vi "MasterAcquisitionFile_DALSA_IOS_MultiWavelength.vi"() -> ()   [LabVIEW 2020]
uses:
  <vilib>/vision/driver/IMAQdx.llb/IMAQdx Acquisition Mode.ctl
  <vilib>/vision/driver/IMAQdx.llb/IMAQdx Camera Control Mode.ctl
  <vilib>/userDefined/High Color/IMAQdx.ctl
  <vilib>/vision/driver/IMAQdx.llb/IMAQdx Buffer Number Mode.ctl
  <vilib>/DAQmx/write.llb/DAQmx Write (Digital 1D Wfm NChan NSamp).vi
  <vilib>/DAQmx/write.llb/DAQmx Write (Digital Bool 1Line 1Point).vi
  <vilib>/DAQmx/read.llb/DAQmx Read (Analog 1D Wfm NChan NSamp).vi
  <vilib>/Waveform/DWDTOps.llb/DWDT Digital to Boolean Array.vi
  <vilib>/DAQmx/create/channels.llb/DAQmx Create Channel (CO-Pulse Generation-Frequency).vi
  <vilib>/DAQmx/configure/timing.llb/DAQmx Timing (Implicit).vi
  <vilib>/DAQmx/create/channels.llb/DAQmx Create Channel (AI-Voltage-Basic).vi
  <vilib>/DAQmx/configure/timing.llb/DAQmx Timing (Sample Clock).vi
  <vilib>/DAQmx/configure/trigger.llb/DAQmx Start Trigger (Digital Edge).vi
  <vilib>/DAQmx/create/channels.llb/DAQmx Create Channel (DO-Digital Output).vi
  <vilib>/Waveform/DWDTOps.llb/DWDT Boolean Array to Digital.vi
  <vilib>/Waveform/DWDTOps.llb/DWDT Uncompress Digital.vi
  <vilib>/DAQmx/miscellaneous.llb/DAQmx Fill In Error Info.vi
  <vilib>/vision/driver/NI_Vision_Acquisition_Software.lvlib
  <resource>/objmgr/imaqdx.rc
  <resource>/objmgr/daqmx.rc
panel:
  out "LED":bool
  out "Auditory":bool
  out "RPad":bool
  out "LPad":bool
  out "Finished":bool
  in  "Generate Stimuli":bool=TRUE
  in  "Sol Stim Parameters":cluster{"Fs":dbl, "Samples":dbl}
  in  "LED Stim Parameters":cluster{"Fs":dbl, "Samples":dbl}
  in  "Sol Duty Cycle (%)":dbl=50.0
  in  "Sol Freq":dbl=1.0
  in  "Sol Dur (s)":dbl=1.0
  in  "LED Duty Cycle (%)":dbl=10.0
  in  "LED Freq":dbl=10.0
  in  "LED Dur (s)":dbl=2.0
  out "Stimulus Order":digitalwaveform[](graph)=[{"t0"=timestamp(0 s since 1904-01-01), "dt"=5e-05, "Y"={"transitions"=[], "data"=array18001000x1[18001000 elements]}}, {"t0"=timestamp(0 s since 1904-01-01), "dt"=5e-05, "Y"={"transitions"=[], "data"=array18001000x1[18001000 elements]}}, {"t0"=timestamp(0 s since 1904-01-01), "dt"=5e-05, "Y"={"transitions"=[], "data"=array18001000x1[18001000 elements]}}, {"t0"=timestamp(0 s since 1904-01-01), "dt"=5e-05, "Y"={"transitions"=[], "data"=array18001000x1[18001000 elements]}}]
  out "Solenoid Stim":digitalwaveform(graph)={"t0"=timestamp(0 s since 1904-01-01), "dt"=5e-05, "Y"={"transitions"=[], "data"=array100000x1[100000 elements]}}
  in  "Trial Offset (s)":dbl=15.0
  in  "Interstim (s)":dbl=30.0
  in  "Right Pad":dbl=1.0
  in  "Left Pad":dbl=1.0
  in  "Auditory":dbl=1.0
  in  "LED":dbl
  out "?":T1(plugin-control)
  out "?":T1(plugin-control)
  out "?":T1(plugin-control)
  out "?":T1(plugin-control)
  in  "stop":bool
  out "CBV Cam":bool
  out "Pupil Cam":bool
  out "Whisk Cam":bool
  out "Web Cam":bool
  out "Analog":bool
  out "Web Cam Fs":dbl(knob) scale=0.0..200.0
  out "CBV Cam Fs":dbl(knob) scale=0.0..200.0
  out "Whisk Cam Fs":dbl(knob) scale=0.0..200.0
  out "Last Whisk\nBuffer 2":u32=1590
  out "Pupil Cam Fs":dbl(knob) scale=0.0..200.0
  out "Dropped 2":u32(slide) caption="Pupil Cam" scale=0.0..99.0
  out "Dev1 Samples":i32
  in  "Dev1 Analog Channels":string[](array[string])=["Cortical_LH", "Force_Sensor", "LPadSol", "RPadSol", "AudSol", "Hippocampus", "EMG", "Cortical_RH", "OptoLED"]
  in  "Analog Acquisition":cluster{"Analog Fs":u16}={"Analog Fs"=20000} {"Analog Fs" format="%0.0f"}
  in  "Sampling Rates":T2={"Web Cam Fs"=30, "Whisk Cam Fs"=150, "Pupil Cam Fs"=30, "CBV Cam Fs"=30}
  out "Notes Size":i32=8
  out "Notes Reversed":string[](array[string])=["Experimenter", "Animal ID", "Hemisphere", "Solenoid PSI", "Isoflurane time", "Session ID", "Amplifier Gain", "LED power (mW)"]
  out "Notes Array":string[](array[string])=["LED power (mW)", "Amplifier Gain", "Session ID", "Isoflurane time", "Solenoid PSI", "Hemisphere", "Animal ID", "Experimenter"]
  in  "Notes:":T3={"Experimenter"="Kevin", "Animal ID"="T305", "Hemisphere"="Both", "Solenoid PSI"="10", "Isoflurane time"="1325", "Session ID"="Imaging Session Four", "Amplifier Gain"="10000", "LED power (mW)"="10"}
  in  "Target Path":path=path "D:/SG06/Imaging Session 4 - 28 July 2022" caption="Final Save Location"
  out "Dropped":u32(slide) caption="Whisk Cam" scale=0.0..999.0
  out "Filename":string="220728_13_37_51"
  out "CBV Camera":bool
  out "Time Elapsed (Min)":cluster{dbl, dbl}(slide)={15.0, 0.0} scale=0.0..15.0 scale format="%#_2g"
  in  "Time (min)":dbl(knob)=15.0 min=0.5 max=20.0 step=0.5 scale=0.0..20.0 scale format="%#_2g"
  in  "Temp Path":path=path "D:/LabVIEW Streamed Data" caption="Temporary Path for Streamed Data"
  out "Last CBV\nBuffer":i32=1590
  out "Last Whisk\nBuffer":u32=7953
  # "Dropped Frames"
  # "Stimuli"
  # "LPAD"
  # "RPAD"
  # "AUD"
  # "LED"
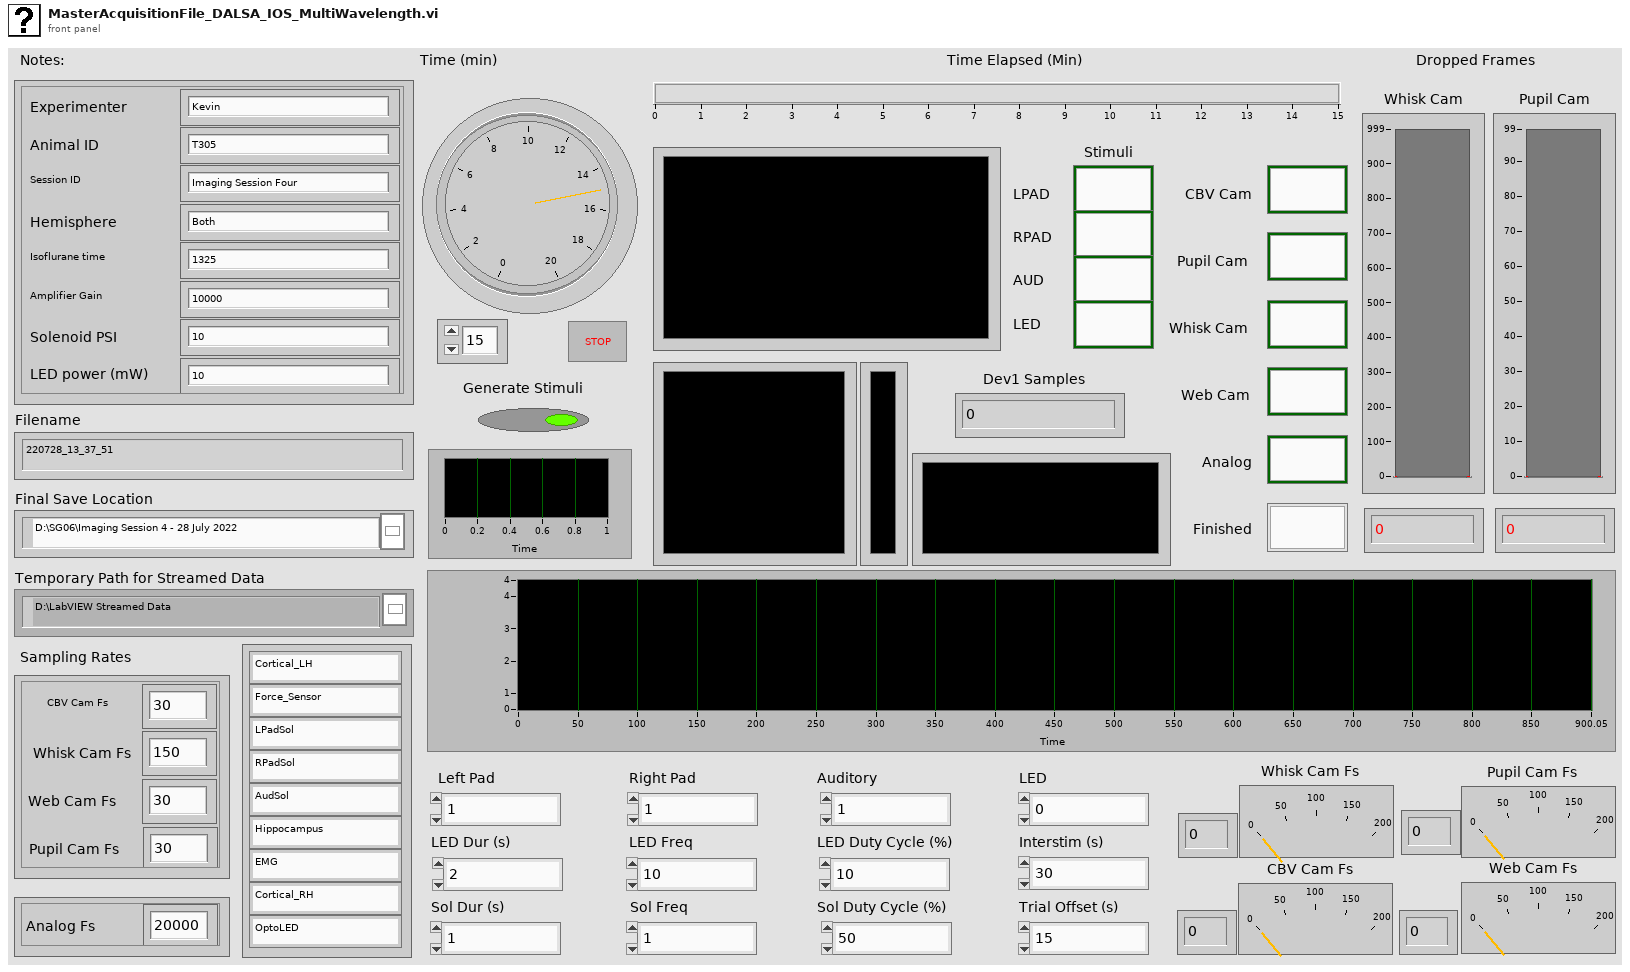
[diagram p1: front panel]
types:
  T1 = typedef "IMAQ Image.ctl" = refnum<image>
  T2 = cluster{"Web Cam Fs":u16, "Whisk Cam Fs":u16, "Pupil Cam Fs":u16, "CBV Cam Fs":u16}
  T3 = cluster{"Experimenter":string, "Animal ID":string, "Hemisphere":string, "Solenoid PSI":string, "Isoflurane time":string, "Session ID":string, "Amplifier Gain":string, "LED power (mW)":string}
  T4 = typedef "IMAQdx.ctl" = refnum<k21>
  T5 = enum16{"open", "replace", "create", "open or create", "replace or create", "replace or create with confirmation"}
  T6 = typedef "Image Type" = u32
  T7 = typedef "NI_Vision_Acquisition_Software.lvlib/IMAQdx Acquisition Mode.ctl" = enum32{"One Shot", "Continuous"}
  T8 = typedef "NI_Vision_Acquisition_Software.lvlib/IMAQdx Camera Control Mode.ctl" = enum32{"Controller", "Listener"}
  T9 = enum16{"open", "open or create", "create or replace", "create", "open (read-only)"}
  T10 = typedef "IMAQ AVI2 Refnum.ctl" = refnum<k20>
  T11 = enum16{"big-endian, network order", "native, host order", "little-endian"}
  T12 = typedef "NI_Vision_Acquisition_Software.lvlib/IMAQdx Buffer Number Mode.ctl" = enum32{"Next", "Last", "Buffer Number", "Every", "Last New"}
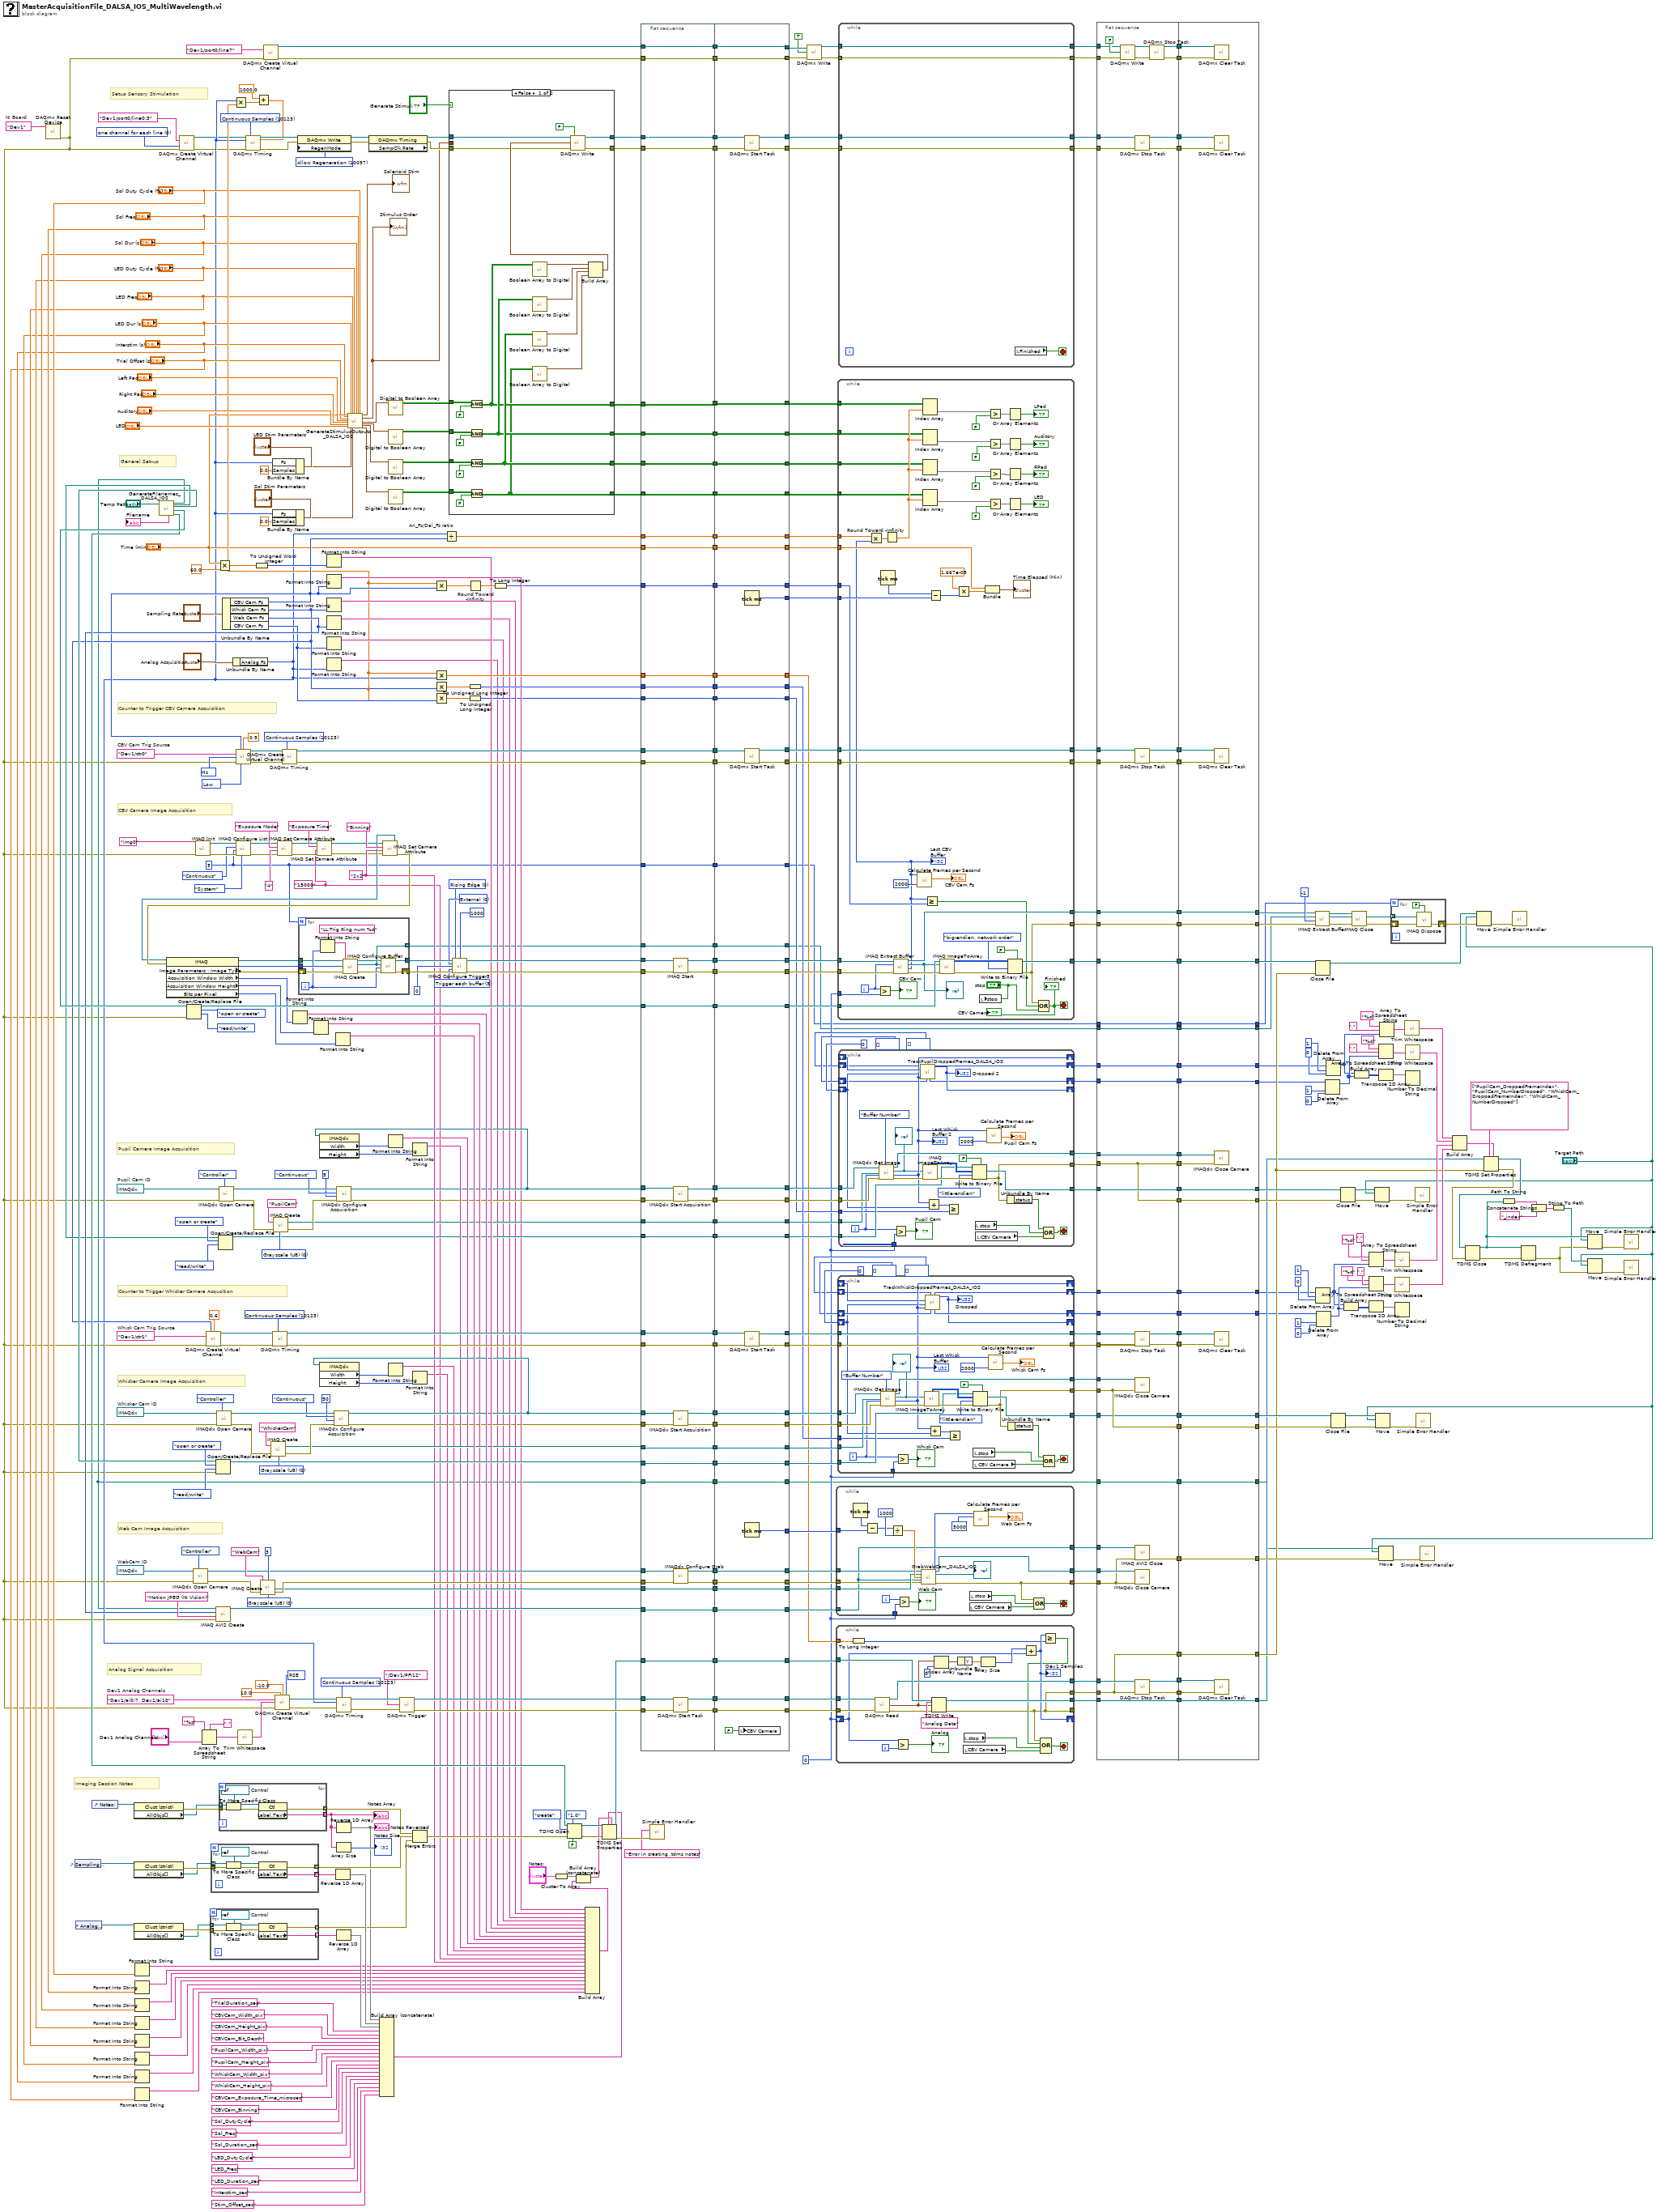
[diagram p0: block diagram]
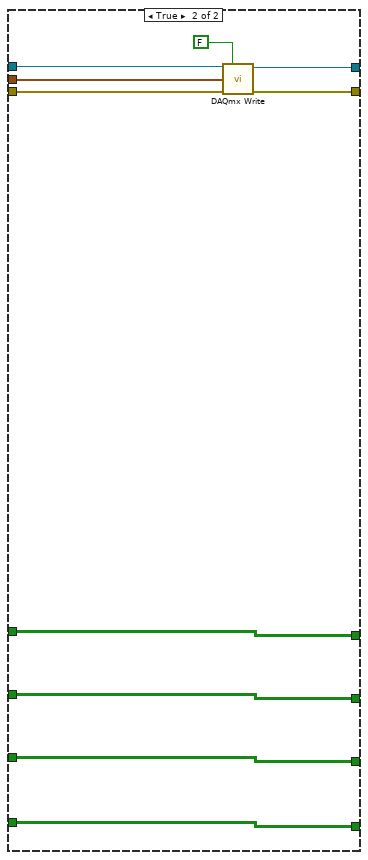
[diagram p2: hidden frame]
diagram:
  w2 = "15000" ("Exposure Time (microsec)")
  w129 = 10097 items=["Allow Regeneration"=10097, "Do Not Allow Regeneration"=10158] ("RegenMode")
  w130 = 10123 items=["Finite Samples"=10178, "Continuous Samples"=10123, "Hardware Timed Single Point"=12522] ("sample mode")
  w133 = 0 items=["one channel for each line", "one channel for all lines"] ("line grouping")
  w327 = tag "Dev1/ai0:7, Dev1/ai10"  # Dev1 Analog Channels
  w330 = T4 "cam3"  # WebCam ID
  w308 = T4 "cam1"  # Whisker Cam ID
  w484 = tag "Dev1/ctr1"  # Whisk Cam Trig Source
  w258 = T4 "cam2"  # Pupil Cam ID
  w95 = tag "Dev1/ctr0"  # CBV Cam Trig Source
  w261 = T6 0 items=["Grayscale (U8)", "Grayscale (I16)", "Grayscale (SGL)", "Complex (CSG)", "RGB (U32)", "HSL (U32)", "RGB (U64)", "Grayscale (U16)"] ("Image Type")
  w248 = "2x2" ("Attribute Value")
  w186 = 0
  w403 = 10123 items=["Finite Samples"=10178, "Continuous Samples"=10123, "Hardware Timed Single Point"=12522] ("sample mode")
  w406 = 10083 items=["default"=-1, "RSE"=10083, "NRSE"=10078, "Differential"=10106, "Pseudodifferential"=12529] ("input terminal configuration")
  w450 = T6 0 items=["Grayscale (U8)", "Grayscale (I16)", "Grayscale (SGL)", "Complex (CSG)", "RGB (U32)", "HSL (U32)", "RGB (U64)", "Grayscale (U16)"] ("Image Type")
  w466 = u32 0 items=["Rising Edge", "Falling Edge"] ("Trigger Polarity")
  w469 = u32 0 items=["External"=0, "RTSI"=1, "ISO In"=2, "Scaled Encoder"=5] ("Trigger Type")
  w460 = tag "Dev1"  # NI Board
  w461 = 10123 items=["Finite Samples"=10178, "Continuous Samples"=10123, "Hardware Timed Single Point"=12522] ("sample mode")
  w464 = 10373 items=["Hz"=10373] ("units")
  w465 = 10214 items=["High"=10192, "Low"=10214] ("idle state")
  w28 = u32 5 ("Number of Buffers")
  w467 = u32 3 items=["Disabled", "Trigger start of acquisition", "Trigger start of each buffer list", "Trigger each buffer", "Trigger each line (linescan)", "Trigger end of acquisition"] ("Action")
  w480 = 10123 items=["Finite Samples"=10178, "Continuous Samples"=10123, "Hardware Timed Single Point"=12522] ("sample mode")
  w487 = T6 0 items=["Grayscale (U8)", "Grayscale (I16)", "Grayscale (SGL)", "Complex (CSG)", "RGB (U32)", "HSL (U32)", "RGB (U64)", "Grayscale (U16)"] ("Image Type")
  # "General Set-up"
  # "Pupil Camera Image Acquisition"
  # "Whisker Camera Image Acquisition"
  # "Imaging Session Notes"
  # "Setup Sensory Stimulation"
  # "CBV Camera Image Acquisition"
  # "Counter to Trigger CBV Camera Acquisition"
  # "Counter to Trigger Whisker Camera Acqusition"
  # "Web Cam Image Acquisition"
  # "Analog Signal Acquisition"
  n1 = call <vilib>:"DAQmx Reset Device.vi"("device in"=w460) -> ("error out"=w20:errorcluster)  [unwired: 14 in]
  n2 = control-ref of="Sampling Rates"() -> (w336:refnum<vi>)
  n3 = control-ref of="Analog Acquisition"() -> (w335:refnum<vi>)
  n4 = control-ref of="Notes:"() -> (w357:refnum<vi>)
  n5 = property class="Clust (strict)"(reference=w357) -> (error out=w360:errorcluster, "AllObjs[]"=w277:refnum<vi>[])  [unwired: 1 in, 1 out]
  n6 = property class="Clust (strict)"(reference=w336) -> (error out=w355:errorcluster, "AllObjs[]"=w278:refnum<vi>[])  [unwired: 1 in, 1 out]
  n7 = property class="Clust (strict)"(reference=w335) -> (error out=w334:errorcluster, "AllObjs[]"=w276:refnum<vi>[])  [unwired: 1 in, 1 out]
  n8 = Format Into String("Sol Duty Cycle (%)") -> (resulting string=w163:string)  [unwired: 3 in, 1 out]
  n9 = Format Into String("Sol Freq") -> (resulting string=w162:string)  [unwired: 3 in, 1 out]
  n10 = Format Into String("Sol Dur (s)") -> (resulting string=w161:string)  [unwired: 3 in, 1 out]
  n11 = Format Into String("LED Duty Cycle (%)") -> (resulting string=w160:string)  [unwired: 3 in, 1 out]
  n12 = Format Into String("LED Freq") -> (resulting string=w159:string)  [unwired: 3 in, 1 out]
  n13 = Format Into String("LED Dur (s)") -> (resulting string=w158:string)  [unwired: 3 in, 1 out]
  n14 = Format Into String("Interstim (s)") -> (resulting string=w157:string)  [unwired: 3 in, 1 out]
  n15 = Format Into String("Trial Offset (s)") -> (resulting string=w156:string)  [unwired: 3 in, 1 out]
  n16 = call "GenerateFilenames_DALSA_IOS.vi"("path"="Temp Path") -> ("TDMS Path"=w352:path, "Dalsa Path"=w457:path, "Basler Path"=w453:path, "WebCam Path"=w22:path, "Analog file name"=→"Filename":string, "Basler2 Path"=w257:path)  [unwired: 3 in, 2 out]
  n17 = call-poly <vilib>:"DAQmx Create Virtual Channel.vi"("lines"=tag "Dev1/port0/line0:3", "line grouping"=w133, "error in"=w20) -> ("task out"=w132:refnum<k21>, "error out"=w131:errorcluster)  [unwired: 11 in]
  n18 = Open/Create/Replace File(file path (use dialog)=w457, error in=w20, operation (0:open)=T5."open or create", access (0:read/write)=enum16{"read/write", "read-only", "write-only"}."read/write") -> (refnum out=w407:refnum<file>)  [unwired: 2 in, 2 out]
  n19 = call <vilib>:"IMAQdx Open Camera.vi"("Camera Control Mode"=IMAQdx_Camera_Control_Mode."Controller", "error in"=w20, "Session In"=w330) -> ("error out"=w446:errorcluster, "Session Out"=w444:T4)  [unwired: 7 in]
  n20 = call <vilib>:"IMAQ Init.vi"("error in (no error)"=w20, "Interface Name"="img0") -> ("error out"=w478:errorcluster, "IMAQ Session Out"=w479:refnum<k11>)  [unwired: 8 out]
  n21 = Array To Spreadsheet String(delimiter (Tab)=",", array="Dev1 Analog Channels", 3:"%s" ("format string")) -> (spreadsheet string=w324:string)
  n22 = for {
    tunnel: [w499] -> w332 mode=indexing
    tunnel: w334 -> [w498]
    tunnel: [w496] -> w333 mode=indexing
    tunnel: w276 -> [w495] mode=indexing
    w500 = refnum<vi> refnum  # Control
    n23 = To More Specific Class(target class=w500, reference=w495, error in=w498) -> (specific class reference=w501:refnum<vi>, error out=w497:errorcluster)
    n24 = property class="Ctl"(reference=w501, error in=w497) -> (error out=w496:errorcluster, "Label.Text"=w499:string)  [unwired: 1 out]
  }
  n25 = for {
    tunnel: [w506] -> w356 mode=indexing
    tunnel: w355 -> [w505]
    tunnel: [w503] -> w342 mode=indexing
    tunnel: w278 -> [w502] mode=indexing
    w507 = refnum<vi> refnum  # Control
    n26 = To More Specific Class(target class=w507, reference=w502, error in=w505) -> (specific class reference=w508:refnum<vi>, error out=w504:errorcluster)
    n27 = property class="Ctl"(reference=w508, error in=w504) -> (error out=w503:errorcluster, "Label.Text"=w506:string)  [unwired: 1 out]
  }
  n28 = Open/Create/Replace File(file path (use dialog)=w453, error in=w20, operation (0:open)=T5."open or create", access (0:read/write)=enum16{"read/write", "read-only", "write-only"}."read/write") -> (refnum out=w423:refnum<file>)  [unwired: 2 in, 2 out]
  n29 = call <vilib>:"IMAQdx Open Camera.vi"("Camera Control Mode"=IMAQdx_Camera_Control_Mode."Controller", "error in"=w20, "Session In"=w308) -> ("error out"=w490:errorcluster, "Session Out"=w493:T4)  [unwired: 7 in]
  n30 = Multiply(x="Time (min)", y=60.0) -> (x*y=w173:dbl)
  n31 = Open/Create/Replace File(file path (use dialog)=w257, operation (0:open)=T5."open or create", access (0:read/write)=enum16{"read/write", "read-only", "write-only"}."read/write") -> (refnum out=w239:refnum<file>)  [unwired: 3 in, 2 out]
  n32 = call <vilib>:"IMAQdx Open Camera.vi"("Camera Control Mode"=IMAQdx_Camera_Control_Mode."Controller", "error in"=w20, "Session In"=w258) -> ("error out"=w264:errorcluster, "Session Out"=w267:T4)  [unwired: 7 in]
  n33 = for {
    tunnel: [w513] -> w359 mode=indexing
    tunnel: w360 -> [w512]
    tunnel: [w510] -> w343 mode=indexing
    tunnel: w277 -> [w509] mode=indexing
    w514 = refnum<vi> refnum  # Control
    n34 = To More Specific Class(target class=w514, reference=w509, error in=w512) -> (specific class reference=w515:refnum<vi>, error out=w511:errorcluster)
    n35 = property class="Ctl"(reference=w515, error in=w511) -> (error out=w510:errorcluster, "Label.Text"=w513:string)  [unwired: 1 out]
  }
  "Notes Array" <- w359
  n36 = Unbundle By Name("Sampling Rates") -> ("CBV Cam Fs"=w174:u16, "Whisk Cam Fs"=w228:u16, "Web Cam Fs"=w329:u16, "CBV Cam Fs"=w222:u16)
  n37 = call-poly <vilib>:"DAQmx Create Virtual Channel.vi"("frequency"=w228, "duty cycle"=0.6, "counter"=w484, "error in"=w20) -> ("task out"=w482:refnum<k21>, "error out"=w481:errorcluster)  [unwired: 10 in]
  n38 = call "IMAQ AVI2 Create"("error in (no error)"=w20, "Codec"="Motion JPEG (NI Vision)", "Frames Per Second"=w329, "AVI Path"=w22) -> ("AVI Refnum"=w436:T10)  [unwired: 6 in, 1 out]
  n39 = Unbundle By Name("Analog Acquisition") -> ("Analog Fs"=w146:u16)
  n40 = Multiply(x=w146, y=w173) -> (x*y=w106:dbl)
  n41 = call-poly <vilib>:"DAQmx Create Virtual Channel.vi"("frequency"=w174, "duty cycle"=0.9, "counter"=w95, "units"=w464, "error in"=w20, "idle state"=w465) -> ("task out"=w463:refnum<k21>, "error out"=w462:errorcluster)  [unwired: 8 in]
  n42 = call <vilib>:"IMAQ Configure List.vi"("Memory Location"=enum16{"System", "Onboard"}."System", "error in (no error)"=w478, "Number of buffers"=w28, "Continuous?"=enum16{"One-Shot", "Continuous"}."Continuous" ("Continuous ?"), "IMAQ Session In"=w479) -> ("error out"=w287:errorcluster, "IMAQ Session Out"=w285:refnum<k11>)  [unwired: 1 in, 4 out]
  n43 = call <vilib>:"Trim Whitespace.vi"("string"=w324) -> ("trimmed string"=w323:string)  [unwired: 1 in]
  n44 = To Unsigned Word Integer(number=w173) -> (unsigned 16bit integer=w319:u16)
  n45 = Add(x=1000.0, y=w106) -> (x+y=w104:dbl)
  n46 = call-poly <vilib>:"DAQmx Timing.vi"("task/channels in"=w132, "sample mode"=w130, "samples per channel"=w104, "rate"=w146, "error in"=w131) -> ("task out"=w126:refnum<k21>, "error out"=w125:errorcluster)  [unwired: 9 in]
  n47 = call "IMAQ Create"("Border Size"=3, "Image Name"="WebCam", "Image Type"=w450, "error in (no error)"=w446) -> ("New Image"=w443:T1, "error out"=w445:errorcluster)  [unwired: 1 in]
  n48 = call-poly <vilib>:"DAQmx Create Virtual Channel.vi"("lines"=tag "Dev1/port0/line7", "error in"=w20) -> ("task out"=w18:refnum<k21>, "error out"=w19:errorcluster)  [unwired: 12 in]
  n49 = call "IMAQ Create"("Image Name"="WhiskerCam", "Image Type"=w487, "error in (no error)"=w490) -> ("New Image"=w306:T1, "error out"=w488:errorcluster)  [unwired: 2 in]
  n50 = Bundle By Name(cluster="LED Stim Parameters", "Fs"=w146, "Samples"=0.0) -> (w179:cluster{"Fs":dbl, "Samples":dbl})
  n51 = Bundle By Name(cluster="Sol Stim Parameters", "Fs"=w146, "Samples"=0.0) -> (w180:cluster{"Fs":dbl, "Samples":dbl})
  n52 = call-poly <vilib>:"DAQmx Timing.vi"("task/channels in"=w482, "sample mode"=w480, "error in"=w481) -> ("task out"=w389:refnum<k21>, "error out"=w387:errorcluster)  [unwired: 11 in]
  n53 = call "IMAQ Create"("Image Name"="PupilCam", "Image Type"=w261, "error in (no error)"=w264) -> ("New Image"=w231:T1, "error out"=w262:errorcluster)  [unwired: 2 in]
  n54 = call-poly <vilib>:"DAQmx Create Virtual Channel.vi"("maximum value"=10.0, "minimum value"=-10.0, "input terminal configuration"=w406, "physical channels"=w327, "name to assign"=w323, "error in"=w20) -> ("task out"=w405:refnum<k21>, "error out"=w404:errorcluster)  [unwired: 8 in]
  n55 = call <vilib>:"IMAQ Set Camera Attribute.vi"("error in (no error)"=w287, "Attribute Value"="4", "Camera Attribute"="Exposure Mode", "IMAQ Session In"=w285) -> ("error out"=w4:errorcluster, "IMAQ Session Out"=w6:refnum<k11>)  [unwired: 4 in]
  n56 = call-poly <vilib>:"DAQmx Timing.vi"("task/channels in"=w463, "sample mode"=w461, "error in"=w462) -> ("task out"=w393:refnum<k21>, "error out"=w391:errorcluster)  [unwired: 11 in]
  n57 = property class="DAQmx Write"(reference=w126, error in=w125, "RegenMode"=w129) -> (reference out=w127:refnum<k21>, error out=w128:errorcluster)
  n58 = call <vilib>:"IMAQ Set Camera Attribute.vi"("error in (no error)"=w4, "Attribute Value"=w2, "Camera Attribute"="Exposure Time", "IMAQ Session In"=w6) -> ("error out"=w3:errorcluster, "IMAQ Session Out"=w5:refnum<k11>)  [unwired: 4 in]
  n59 = Format Into String(w319) -> (resulting string=w321:string)  [unwired: 3 in, 1 out]
  n60 = Format Into String(w174) -> (resulting string=w226:string)  [unwired: 3 in, 1 out]
  n61 = Format Into String(w228) -> (resulting string=w225:string)  [unwired: 3 in, 1 out]
  n62 = Format Into String(w329) -> (resulting string=w224:string)  [unwired: 3 in, 1 out]
  n63 = Format Into String(w222) -> (resulting string=w192:string)  [unwired: 3 in, 1 out]
  n64 = Format Into String(w146) -> (resulting string=w191:string)  [unwired: 3 in, 1 out]
  n65 = call <vilib>:"IMAQdx Configure Acquisition.vi"("error in"=w488, "Number of Buffers"=u32 50, "Continuous?"=IMAQdx_Acquisition_Mode."Continuous", "Session In"=w493) -> ("error out"=w199:errorcluster, "Session Out"=w307:T4)  [unwired: 6 in]
  n66 = property class="IMAQdx"(reference=w307) -> ("Width"=w318:u32, "Height"=w317:u32)  [unwired: 1 in, 2 out]
  n67 = Reverse 1D Array(array=w356) -> (reversed array=w346:string[])
  n68 = Reverse 1D Array(array=w359) -> (reversed array=w275:string[])
  "Notes Reversed" <- w275
  n69 = Array Size(array=w359) -> (size(s)=→"Notes Size":i32)
  n70 = Reverse 1D Array(array=w332) -> (reversed array=w331:string[])
  n71 = call <vilib>:"IMAQdx Configure Acquisition.vi"("error in"=w262, "Number of Buffers"=u32 5, "Continuous?"=IMAQdx_Acquisition_Mode."Continuous", "Session In"=w267) -> ("error out"=w241:errorcluster, "Session Out"=w232:T4)  [unwired: 6 in]
  n72 = property class="IMAQdx"(reference=w232) -> ("Width"=w256:u32, "Height"=w255:u32)  [unwired: 1 in, 2 out]
  n73 = call-poly <vilib>:"DAQmx Timing.vi"("task/channels in"=w405, "sample mode"=w403, "rate"=w146, "error in"=w404) -> ("task out"=w274:refnum<k21>, "error out"=w402:errorcluster)  [unwired: 10 in]
  n74 = call "GenerateStimulusOutputs_DALSA_IOS.vi"("Trial duration (min)"="Time (min)", "Rest duration(s)"="Interstim (s)", "trial offset (s)"="Trial Offset (s)", "Left Pad"="Left Pad", "Right Pad"="Right Pad", "Auditory"="Auditory", "LED"="LED", "LED Stim Duration (s)"="LED Dur (s)", "LED Stim Parameters"=w179, "LED Frequency"="LED Freq", "Sol Stim Parameters"=w180, "LED duty cycle (%)"="LED Duty Cycle (%)", "Sol Stim Duration (s)"="Sol Dur (s)", "Sol Frequency"="Sol Freq", "Sol Duty Cycle (%)"="Sol Duty Cycle (%)") -> ("Solenoid Stim Waveforms"=→"Solenoid Stim":digitalwaveform, "Stimulus Digital Outputs"=w107:digitalwaveform[], "Left Pad Out"=w137:digitalwaveform, "Auditory Out"=w136:digitalwaveform, "Right Pad Out"=w135:digitalwaveform, "LED Out"=w134:digitalwaveform)  [unwired: 7 in]
  "Stimulus Order" <- w107
  n75 = property class="DAQmx Timing" props=["SampClk.Rate"](reference=w127, error in=w128) -> (reference out=w123:refnum<k21>, error out=w122:errorcluster)  [unwired: 1 out]
  n76 = Build Array (concatenate)(w275, w346, w331, "TrialDuration_sec", "CBVCam_Width_pix", "CBVCam_Height_pix", "CBVCam_Bit_Depth", "PupilCam_Width_pix", "PupilCam_Height_pix", "WhiskCam_Width_pix", "WhiskCam_Height_pix", "CBVCam_Exposure_Time_microsec" ("element"), "CBVCam_Binning" ("element"), "Sol_DutyCycle", "Sol_Freq", "Sol_Duration_sec", "LED_DutyCycle", "LED_Freq", "LED_Duration_sec", "Interstim_sec", "Stim_Offset_sec") -> (w269:string[])
  n77 = call <vilib>:"IMAQ Set Camera Attribute.vi"("error in (no error)"=w3, "Attribute Value"=w248, "Camera Attribute"="Binning", "IMAQ Session In"=w5) -> ("error out"=w286:errorcluster, "IMAQ Session Out"=w284:refnum<k11>)  [unwired: 4 in]
  n78 = property class="IMAQ"(reference=w284, error in=w286) -> (reference out=w293:refnum<k11>, error out=w292:errorcluster, "Image Parameters : Image Type"=w474:u32, "Acquisition Window Width"=w316:u32, "Acquisition Window Height"=w315:u32, "Bits per Pixel"=w314:u32)
  n79 = Format Into String(w316) -> (resulting string=w313:string)  [unwired: 3 in, 1 out]
  n80 = for {
    N: w28 -> [_]
    tunnel: [w525] -> w471
    tunnel: w474 -> [w523]
    shift-right: [w524] -> w470
    shift-left: w292 -> [w522]
    tunnel: [w517] -> w33 mode=indexing
    tunnel: w293 -> [w516]
    i -> [w518]
    n81 = Format Into String(format string="LL Trig Ring num %d", w518) -> (resulting string=w520:string)  [unwired: 2 in, 1 out]
    n82 = call "IMAQ Create"("Image Name"=w520, "Image Type"=w523, "error in (no error)"=w522) -> ("New Image"=w517:T1, "error out"=w521:errorcluster)  [unwired: 1 in, 1 out]
    n83 = call <vilib>:"IMAQ Configure Buffer.vi"("error in (no error)"=w521, "Buffer Number"=w518, "Image In"=w517, "IMAQ Session In"=w516) -> ("error out"=w524:errorcluster, "IMAQ Session Out"=w525:refnum<k11>)  [unwired: 2 in, 4 out]
  }
  n84 = Format Into String(w315) -> (resulting string=w271:string)  [unwired: 3 in, 1 out]
  n85 = Format Into String(w314) -> (resulting string=w312:string)  [unwired: 3 in, 1 out]
  n86 = Format Into String(w256) -> (resulting string=w244:string)  [unwired: 3 in, 1 out]
  n87 = Format Into String(w318) -> (resulting string=w246:string)  [unwired: 3 in, 1 out]
  n88 = call-poly <vilib>:"Digital to Boolean Array.vi"("digital waveform"=w137) -> ("boolean array"=w115:bool[][])  [unwired: 9 in, 1 out]
  n89 = call-poly <vilib>:"Digital to Boolean Array.vi"("digital waveform"=w136) -> ("boolean array"=w114:bool[][])  [unwired: 9 in, 1 out]
  n90 = call-poly <vilib>:"Digital to Boolean Array.vi"("digital waveform"=w135) -> ("boolean array"=w113:bool[][])  [unwired: 9 in, 1 out]
  n91 = call-poly <vilib>:"Digital to Boolean Array.vi"("digital waveform"=w134) -> ("boolean array"=w112:bool[][])  [unwired: 9 in, 1 out]
  n92 = call-poly <vilib>:"DAQmx Trigger.vi"("task/channels in"=w274, "source"=tag "/Dev1/PFI12", "error in"=w402) -> ("task out"=w401:refnum<k21>, "error out"=w400:errorcluster)  [unwired: 11 in]
  n93 = Format Into String(w255) -> (resulting string=w245:string)  [unwired: 3 in, 1 out]
  n94 = Format Into String(w317) -> (resulting string=w247:string)  [unwired: 3 in, 1 out]
  n95 = Merge Errors(w343, w342, w333) -> (w341:errorcluster)
  n96 = Multiply(x=w173, y=w174) -> (x*y=w455:dbl)
  n97 = Multiply(x=w173, y=w146) -> (x*y=w297:dbl)
  n98 = Multiply(x=w228, y=w173) -> (x*y=w272:dbl)
  n99 = Multiply(x=w222, y=w173) -> (x*y=w227:dbl)
  n100 = Divide "An_Fs/Dal_Fs ratio"(x=w146, y=w174) -> (x/y=w90:dbl)
  n101 = case shown="False" "Generate Stimuli" {
    tunnel: w123 -> [w536 w557]
    tunnel: w122 -> [w535 w556]
    tunnel: [w533 w555] -> w120
    tunnel: [w534 w554] -> w118
    tunnel: w115 -> [w544 w553]
    tunnel: w114 -> [w545 w552]
    tunnel: w113 -> [w546 w551]
    tunnel: w112 -> [w547 w550]
    tunnel: [w528 w553] -> w111
    tunnel: [w529 w552] -> w110
    tunnel: [w530 w551] -> w109
    tunnel: [w526 w550] -> w108
    tunnel: w107 -> [_ w549]
    frame False {
      n102 = Compound Arithmetic op=AND(w544, FALSE) -> (w528:bool[][])
      n103 = Compound Arithmetic op=AND(w545, FALSE) -> (w529:bool[][])
      n104 = Compound Arithmetic op=AND(w546, FALSE) -> (w530:bool[][])
      n105 = Compound Arithmetic op=AND(w547, FALSE) -> (w526:bool[][])
      n106 = call-poly <vilib>:"Boolean Array to Digital.vi"("boolean array"=w528) -> ("digital waveform"=w538:digitalwaveform)  [unwired: 9 in, 1 out]
      n107 = call-poly <vilib>:"Boolean Array to Digital.vi"("boolean array"=w529) -> ("digital waveform"=w532:digitalwaveform)  [unwired: 9 in, 1 out]
      n108 = call-poly <vilib>:"Boolean Array to Digital.vi"("boolean array"=w530) -> ("digital waveform"=w531:digitalwaveform)  [unwired: 9 in, 1 out]
      n109 = call-poly <vilib>:"Boolean Array to Digital.vi"("boolean array"=w526) -> ("digital waveform"=w527:digitalwaveform)  [unwired: 9 in, 1 out]
      n110 = Build Array(w538, w532, w531, w527) -> (w537:digitalwaveform[])
      n111 = call-poly <vilib>:"DAQmx Write.vi"("task/channels in"=w536, "auto start"=FALSE, "data"=w537, "error in"=w535) -> ("task out"=w533:refnum<k21>, "error out"=w534:errorcluster)  [unwired: 9 in, 1 out]
    }
    frame True {
      n112 = call-poly <vilib>:"DAQmx Write.vi"("task/channels in"=w557, "auto start"=FALSE, "data"=w549, "error in"=w556) -> ("task out"=w555:refnum<k21>, "error out"=w554:errorcluster)  [unwired: 9 in, 1 out]
    }
  }
  n113 = call <vilib>:"IMAQ Configure Trigger3.vi"("IMAQ Session In"=w471, "Polarity"=w466, "Frame timeout (ms)"=u32 1000 ("Frame Timeout (ms)"), "Type"=w469, "Line Number"=u32 0 ("Trigger Line Number"), "Action"=w467, "error in (no error)"=w470) -> ("IMAQ Session Out"=w422:refnum<k11>, "error out"=w421:errorcluster)  [unwired: 2 in, 5 out]
  n114 = To Unsigned Long Integer(number=w272) -> (unsigned 32bit integer=w295:u32)
  n115 = To Unsigned Long Integer(number=w227) -> (unsigned 32bit integer=w223:u32)
  n116 = Round Toward -Infinity(1:w455) -> (0:w454:dbl)
  n117 = To Long Integer(number=w454) -> (32bit integer=w200:i32)
  n118 = Cluster To Array(cluster="Notes:") -> (array=w353:string[])
  n119 = TDMS Open(6:FALSE ("disable buffering? (T)"), 7:enum16{"1.0", "2.0"}."1.0" ("file format version (2.0)"), 8:w341, 10:T9."create" ("operation (0:open)"), 11:w352) -> (0:w347:errorcluster, 3:w348:refnum<k34>)  [unwired: 2 in]
  n120 = Build Array(w226, w225, w224, w192, w191, w321, w313, w271, w312, w244, w245, w246, w247, w2, w248, w163, w162, w161, w160, w159, w158, w157, w156) -> (w328:string[])
  n121 = Build Array (concatenate)(w353, w328) -> (w345:string[])
  n122 = TDMS Set Properties(5:w345, 7:w269, 8:w347, 11:w348) -> (0:w340:errorcluster, 3:w344:refnum<k34>)  [unwired: 2 in, 2 out]
  n123 = flat-sequence {
    tunnel: w445 -> [w606]
    tunnel: w444 -> [w605]
    tunnel: w443 -> [w604]
    tunnel: [w604] -> w442
    tunnel: [w603] -> w440
    tunnel: [w602] -> w438
    tunnel: w436 -> [w601]
    tunnel: [w601] -> w435
    tunnel: w307 -> [w600]
    tunnel: w199 -> [w599]
    tunnel: [w598] -> w430
    tunnel: [w597] -> w428
    tunnel: [w596] -> w426
    tunnel: w306 -> [w596]
    tunnel: [w595] -> w424
    tunnel: w423 -> [w595]
    tunnel: w422 -> [w594]
    tunnel: w421 -> [w593]
    tunnel: [w592] -> w419
    tunnel: [w591] -> w417
    tunnel: w200 -> [w590]
    tunnel: [w590] -> w413
    tunnel: "Time (min)" -> [w589]
    tunnel: [w589] -> w410
    tunnel: [w588] -> w408
    tunnel: w407 -> [w588]
    tunnel: w401 -> [w587]
    tunnel: w400 -> [w586]
    tunnel: [w585] -> w399
    tunnel: [w584] -> w398
    tunnel: [w583] -> w394
    tunnel: w344 -> [w583]
    tunnel: w393 -> [w582]
    tunnel: [w582] -> w392
    tunnel: w391 -> [w581]
    tunnel: [w581] -> w390
    tunnel: w389 -> [w580]
    tunnel: [w580] -> w388
    tunnel: w387 -> [w579]
    tunnel: [w579] -> w386
    tunnel: w297 -> [w578]
    tunnel: [w578] -> w296
    tunnel: w295 -> [w577]
    tunnel: [w577] -> w294
    tunnel: [w572] -> w243
    tunnel: w232 -> [w573]
    tunnel: [w570] -> w242
    tunnel: w241 -> [w571]
    tunnel: [w576] -> w240
    tunnel: w239 -> [w576]
    tunnel: w231 -> [w575]
    tunnel: [w575] -> w230
    tunnel: w223 -> [w574]
    tunnel: [w574] -> w221
    tunnel: [w569] -> w145
    tunnel: w111 -> [w569]
    tunnel: [w568] -> w144
    tunnel: w110 -> [w568]
    tunnel: [w567] -> w143
    tunnel: w109 -> [w567]
    tunnel: [w566] -> w142
    tunnel: w108 -> [w566]
    tunnel: [w565] -> w121
    tunnel: w120 -> [w565]
    tunnel: [w564] -> w119
    tunnel: w118 -> [w564]
    tunnel: w90 -> [w563]
    tunnel: [w563] -> w89
    tunnel: w33 -> [w562]
    tunnel: [w562] -> w36
    tunnel: w28 -> [w561]
    tunnel: [w561] -> w31
    tunnel: w22 -> [w560]
    tunnel: [w560] -> w23
    tunnel: w19 -> [w558]
    tunnel: w18 -> [w559]
    tunnel: [w559] -> w16
    tunnel: [w558] -> w14
    tunnel: [w654] -> w447
    tunnel: w442 -> [w653]
    tunnel: [w653] -> w441
    tunnel: w440 -> [w652]
    tunnel: [w652] -> w439
    tunnel: w438 -> [w651]
    tunnel: [w651] -> w437
    tunnel: w435 -> [w650]
    tunnel: [w650] -> w434
    tunnel: [w632] -> w433
    tunnel: [w631] -> w432
    tunnel: [w649] -> w431
    tunnel: w430 -> [w649]
    tunnel: [w648] -> w429
    tunnel: w428 -> [w648]
    tunnel: [w647] -> w427
    tunnel: w426 -> [w647]
    tunnel: [w646] -> w425
    tunnel: w424 -> [w646]
    tunnel: [w645] -> w420
    tunnel: w419 -> [w645]
    tunnel: [w644] -> w418
    tunnel: w417 -> [w644]
    tunnel: [w636] -> w416
    tunnel: [w635] -> w415
    tunnel: [w643] -> w414
    tunnel: w413 -> [w642]
    tunnel: [w642] -> w412
    tunnel: [w641] -> w411
    tunnel: w410 -> [w641]
    tunnel: [w640] -> w409
    tunnel: w408 -> [w640]
    tunnel: [w639] -> w396
    tunnel: w399 -> [w639]
    tunnel: [w638] -> w397
    tunnel: w398 -> [w638]
    tunnel: [w637] -> w189
    tunnel: w394 -> [w637]
    tunnel: w392 -> [w634]
    tunnel: w390 -> [w633]
    tunnel: w388 -> [w630]
    tunnel: w386 -> [w629]
    tunnel: w296 -> [w628]
    tunnel: [w628] -> w190
    tunnel: w294 -> [w627]
    tunnel: [w627] -> w220
    tunnel: w243 -> [w625]
    tunnel: w242 -> [w624]
    tunnel: w240 -> [w623]
    tunnel: [w625] -> w235
    tunnel: [w624] -> w234
    tunnel: [w623] -> w233
    tunnel: [w622] -> w229
    tunnel: w230 -> [w622]
    tunnel: [w621] -> w219
    tunnel: w221 -> [w621]
    tunnel: w145 -> [w617]
    tunnel: w144 -> [w620]
    tunnel: w143 -> [w619]
    tunnel: w142 -> [w618]
    tunnel: [w617] -> w141
    tunnel: [w620] -> w140
    tunnel: [w619] -> w139
    tunnel: [w618] -> w138
    tunnel: w121 -> [w616]
    tunnel: w119 -> [w615]
    tunnel: [w614] -> w117
    tunnel: [w613] -> w116
    tunnel: w89 -> [w612]
    tunnel: [w612] -> w88
    tunnel: w36 -> [w611]
    tunnel: [w611] -> w35
    tunnel: w31 -> [w610]
    tunnel: [w610] -> w30
    tunnel: [w609] -> w25
    tunnel: w23 -> [w609]
    tunnel: [w608] -> w17
    tunnel: w16 -> [w608]
    tunnel: [w607] -> w15
    tunnel: w14 -> [w607]
    frame #0 {
      n124 = call <vilib>:"IMAQ Start.vi"("error in (no error)"=w593, "IMAQ Session In"=w594) -> ("error out"=w591:errorcluster, "IMAQ Session Out"=w592:refnum<k11>)  [unwired: 8 out]
      n125 = call <vilib>:"IMAQdx Start Acquisition.vi"("error in"=w571, "Session In"=w573) -> ("error out"=w570:errorcluster, "Session Out"=w572:T4)  [unwired: 8 in]
      n126 = call <vilib>:"IMAQdx Start Acquisition.vi"("error in"=w599, "Session In"=w600) -> ("error out"=w597:errorcluster, "Session Out"=w598:T4)  [unwired: 8 in]
      n127 = call <vilib>:"IMAQdx Configure Grab.vi"("error in"=w606, "Session In"=w605) -> ("error out"=w602:errorcluster, "Session Out"=w603:T4)  [unwired: 8 in]
      n128 = call <vilib>:"DAQmx Start Task.vi"("task/channels in"=w587, "error in"=w586) -> ("task out"=w585:refnum<k21>, "error out"=w584:errorcluster)  [unwired: 12 in]
    }
    frame #1 {
      n129 = local write "CBV Camera"(FALSE ("Finished Acquiring")) -> ()
      n130 = call <vilib>:"DAQmx Start Task.vi"("task/channels in"=w616, "error in"=w615) -> ("task out"=w614:refnum<k21>, "error out"=w613:errorcluster)  [unwired: 12 in]
      n131 = Tick Count (ms)() -> (millisecond timer value=w643:u32)
      n132 = call <vilib>:"DAQmx Start Task.vi"("task/channels in"=w634, "error in"=w633) -> ("task out"=w636:refnum<k21>, "error out"=w635:errorcluster)  [unwired: 12 in]
      n133 = call <vilib>:"DAQmx Start Task.vi"("task/channels in"=w630, "error in"=w629) -> ("task out"=w632:refnum<k21>, "error out"=w631:errorcluster)  [unwired: 12 in]
      n134 = Tick Count (ms)() -> (millisecond timer value=w654:u32)
    }
  }
  n135 = call <vilib>:"Simple Error Handler.vi"("error source (\" \")"="Error in creating .tdms notes" ("error source (\" \")"), "error in (no error)"=w340) -> ()  [unwired: 3 in, 5 out]
  n136 = call-poly <vilib>:"DAQmx Write.vi"("task/channels in"=w17, "data"=TRUE, "error in"=w15) -> ("task out"=w9:refnum<k21>, "error out"=w8:errorcluster)  [unwired: 10 in, 1 out]
  n137 = while {
    tunnel: w397 -> [w677]
    tunnel: w396 -> [w676]
    tunnel: w189 -> [w675]
    tunnel: [w674] -> w56
    tunnel: [w663] -> _
    tunnel: [w673] -> w87
    shift-right: [w667] -> _
    shift-left: w186 -> [w658]
    tunnel: [w663] -> w86
    tunnel: w190 -> [w661]
    i -> [w659]
    stop <- w664 stop-if-true
    n138 = To Long Integer(number=w661) -> (32bit integer=w662:i32)
    n139 = call-poly <vilib>:"DAQmx Read.vi"("task/channels in"=w676, "error in"=w677) -> ("task out"=w673:refnum<k21>, "data"=w655:waveform(dbl)[], "error out"=w666:errorcluster)  [unwired: 11 in]
    n140 = Greater?(x=w658, y=w659) -> (0:→"Analog":bool)
    n141 = TDMS Write(0:w675, 5:"Analog Data" ("group name in (Untitled)"), 9:w655, 11:w666) -> (4:w674:refnum<k34>, 15:w663:errorcluster)  [unwired: 2 in, 2 out]
    n142 = Index Array(array=w655, index=0) -> (element=w670:waveform(dbl))
    n143 = Unbundle By Name(w670) -> ("Y"=w669:dbl[])
    n144 = local read "CBV Camera"() -> (w657:bool)
    n145 = local read "stop"() -> (w656:bool)
    n146 = Array Size(array=w669) -> (size(s)=w668:i32)
    n147 = Add(x=w668, y=w658) -> (x+y=w667:i32)
    "Dev1 Samples" <- w667
    n148 = Greater Or Equal?(x=w667, y=w662) -> (x >= y?=w665:bool)
    n149 = Compound Arithmetic op=OR(w663, w665, w656, w657) -> (w664:bool)
  }
  n150 = while {
    tunnel: w447 -> [w694]
    tunnel: w441 -> [w692]
    tunnel: w439 -> [w691]
    tunnel: w437 -> [w690]
    tunnel: w434 -> [w688]
    tunnel: [w689] -> w78
    tunnel: [w680] -> w79
    tunnel: [w688] -> w77
    tunnel: w186 -> [w683]
    i -> [w684]
    stop <- w681 stop-if-true
    n151 = Tick Count (ms)() -> (millisecond timer value=w696:u32)
    n152 = Subtract(x=w696, y=w694) -> (x-y=w697:u32)
    n153 = Divide(x=w697, y=u32 1000) -> (x/y=w693:dbl)
    n154 = Greater?(x=w684, y=w683) -> (0:→"Web Cam":bool)
    n155 = call "GrabWebCam_DALSA_IOS.vi"("Session In"=w691, "Image In"=w692, "Trial Time"=w693, "AVI Refnum"=w688, "error in"=w690) -> ("Session Out"=w689:T4, "WebCam Img Out"=→"?":T1, "Buffer Number Out"=w687:u32, "error out"=w680:errorcluster)  [unwired: 7 in]
    n156 = local read "CBV Camera"() -> (w682:bool)
    n157 = local read "stop"() -> (w679:bool)
    n158 = call <vilib>:"Calculate Frames per Second.vi"("Update Interval (ms)"=u32 5000, "Buffer Number"=w687) -> ("Processed Frames/s"=→"Web Cam Fs":dbl)  [unwired: 7 in, 2 out]
    n159 = Compound Arithmetic op=OR(w680, w679, w682) -> (w681:bool)
  }
  n160 = while {
    tunnel: w420 -> [w751]
    tunnel: w418 -> [w752]
    tunnel: [w734] -> w39
    tunnel: [w732] -> w42
    tunnel: [w746] -> w67
    tunnel: [w741] -> w99
    tunnel: w416 -> [w741]
    tunnel: [w740] -> w98
    tunnel: w415 -> [w740]
    tunnel: w414 -> [w739]
    tunnel: w412 -> [w738]
    tunnel: w411 -> [w737]
    tunnel: w409 -> [w731]
    tunnel: w186 -> [w726]
    tunnel: w141 -> [w710]
    tunnel: w140 -> [w711]
    tunnel: w139 -> [w705]
    tunnel: w138 -> [w702]
    tunnel: w88 -> [w699]
    i -> [w727]
    stop <- w721 stop-if-true
    n161 = Greater?(x=w727, y=w726) -> (0:→"CBV Cam":bool)
    n162 = Tick Count (ms)() -> (millisecond timer value=w744:u32)
    n163 = call <vilib>:"IMAQ Extract Buffer.vi"("error in (no error)"=w752, "Buffer to extract"=w727, "IMAQ Session In"=w751) -> ("error out"=w745:errorcluster, "Buffer Number"=w722:i32, "Image Out"=w724:T1, "IMAQ Session Out"=w732:refnum<k11>)  [unwired: 5 out]
    "Last CBV\nBuffer" <- w722
    "?" <- w724
    n164 = Multiply(x=w699, y=w722) -> (x*y=w723:dbl)
    n165 = Round Toward -Infinity(1:w723) -> (0:w716:dbl)
    n166 = call <vilib>:"Calculate Frames per Second.vi"("Update Interval (ms)"=u32 2000, "Buffer Number"=w722) -> ("Processed Frames/s"=→"CBV Cam Fs":dbl)  [unwired: 7 in, 2 out]
    n167 = Index Array(array=w710, index (row)=w716) -> (element=w709:bool[])  [unwired: 1 in]
    n168 = Index Array(array=w711, index (row)=w716) -> (element=w707:bool[])  [unwired: 1 in]
    n169 = Index Array(array=w705, index (row)=w716) -> (element=w704:bool[])  [unwired: 1 in]
    n170 = Index Array(array=w702, index (row)=w716) -> (element=w701:bool[])  [unwired: 1 in]
    n171 = Greater Or Equal?(x=w722, y=w738) -> (x >= y?=w730:bool)
    n172 = Subtract(x=w744, y=w739) -> (x-y=w743:u32)
    n173 = call "IMAQ ImageToArray"("error in (no error)"=w745, "Image"=w724) -> ("error out"=w750:errorcluster, "Image Pixels (I16)"=w749:i16[][])  [unwired: 2 in, 3 out]
    n174 = Multiply(x=w743, y=1.667e-05) -> (x*y=w742:dbl)
    n175 = local write "stop"("stop") -> ()
    n176 = Bundle("Time (min)"=w737, w742) -> (→"Time Elapsed (Min)":cluster{"Time (min)":dbl, dbl})  [unwired: 1 in]
    n177 = Greater?(x=w709, y=FALSE ("Boolean")) -> (0:w708:bool[])
    n178 = Greater?(x=w707, y=FALSE ("Boolean")) -> (0:w706:bool[])
    n179 = Greater?(x=w704, y=FALSE ("Boolean")) -> (0:w703:bool[])
    n180 = Greater?(x=w701, y=FALSE ("Boolean")) -> (0:w700:bool[])
    n181 = Or Array Elements(Boolean array=w708) -> (logical OR=→"LPad":bool)
    n182 = Or Array Elements(Boolean array=w706) -> (logical OR=→"Auditory":bool)
    n183 = Or Array Elements(Boolean array=w703) -> (logical OR=→"RPad":bool)
    n184 = Or Array Elements(Boolean array=w700) -> (logical OR=→"LED":bool)
    n185 = Write to Binary File(file (use dialog)=w731, data=w749, error in=w750, 5:FALSE ("prepend array or string size? (T)"), 9:T11."big-endian, network order" ("byte order (0:big-endian, network order)")) -> (refnum out=w746:refnum<file>, error out=w734:errorcluster)  [unwired: 1 in, 1 out]
    n186 = Compound Arithmetic op=OR(w734, w730, "stop") -> (w721:bool)
    "CBV Camera" <- w721
    "Finished" <- w721
  }
  n187 = while {
    tunnel: w433 -> [w779]
    tunnel: [w780] -> w82
    tunnel: w432 -> [w780]
    tunnel: [w779] -> w83
    tunnel: [w772] -> w73
    tunnel: [w773] -> w74
    tunnel: [w778] -> w69
    tunnel: w431 -> [w777]
    tunnel: w429 -> [w776]
    tunnel: w427 -> [w775]
    tunnel: w425 -> [w774]
    shift-right: [w763] -> _
    shift-left: _ -> [w761]
    shift-right: [w758] -> _
    shift-left: u32 0 ("New Lost") -> [w762]
    shift-right: [w759] -> w51
    shift-left: u32[] [] ("NewBuffNum") -> [w760]
    shift-right: [w765] -> w54
    shift-left: u32[] [] ("NewNumLost") -> [w764]
    tunnel: w220 -> [w770]
    tunnel: w186 -> [w766]
    i -> [w753]
    stop <- w769 stop-if-true
    n188 = call <vilib>:"IMAQdx Get Image.vi"("Buffer Number Mode (Next)"=IMAQdx_Buffer_Number_Mode."Buffer Number", "error in"=w776, "Buffer Number In"=w753, "Image In"=w775, "Session In"=w777) -> ("error out"=w786:errorcluster, "Buffer Number Out"=w763:u32, "Image Out"=w755:T1, "Session Out"=w772:T4)  [unwired: 3 in]
    "Last Whisk\nBuffer" <- w763
    "?" <- w755
    n189 = Greater?(x=w753, y=w766) -> (0:→"Whisk Cam":bool)
    n190 = call "IMAQ ImageToArray"("error in (no error)"=w786, "Image"=w755) -> ("error out"=w785:errorcluster, "Image Pixels (U8)"=w784:u8[][])  [unwired: 2 in, 3 out]
    n191 = call "TrackWhiskDroppedFrames_DALSA_IOS.vi"("NumLost"=w764, "BuffNum"=w760, "Curr Buffer"=w763, "Prev Lost"=w762, "Prev Buffer"=w761) -> ("New Lost"=w758:u32, "NewNumLost"=w765:u32[], "NewBuffNum"=w759:u32[])  [unwired: 4 in]
    "Dropped" <- w758
    n192 = Add(x=w763, y=w762) -> (x+y=w771:u32)
    n193 = Greater Or Equal?(x=w771, y=w770) -> ()  [unwired: 1 out]
    n194 = Write to Binary File(file (use dialog)=w774, data=w784, error in=w785, 5:FALSE ("prepend array or string size? (T)"), 9:T11."little-endian" ("byte order (0:big-endian, network order)")) -> (refnum out=w778:refnum<file>, error out=w773:errorcluster)  [unwired: 1 in, 1 out]
    n195 = local read "stop"() -> (w757:bool)
    n196 = local read "CBV Camera"() -> (w756:bool)
    n197 = call <vilib>:"Calculate Frames per Second.vi"("Update Interval (ms)"=u32 2000, "Buffer Number"=w763) -> ("Processed Frames/s"=→"Whisk Cam Fs":dbl)  [unwired: 7 in, 2 out]
    n198 = Unbundle By Name(w773) -> ("status"=w754:bool)
    n199 = Compound Arithmetic op=OR(w754, w757, w756) -> (w769:bool)
  }
  n200 = while {
    tunnel: w117 -> [w790]
    tunnel: [w791] -> w102
    tunnel: w116 -> [w791]
    tunnel: [w790] -> w103
    tunnel: [w789] -> w10
    tunnel: w9 -> [w789]
    tunnel: w8 -> [w788]
    tunnel: [w788] -> w7
    stop <- w792 stop-if-true
    n201 = local read "Finished"() -> (w792:bool)
  }
  n202 = while {
    tunnel: [w807] -> w93
    tunnel: [w808] -> w92
    tunnel: [w817] -> w64
    tunnel: w235 -> [w816]
    tunnel: w234 -> [w815]
    tunnel: w229 -> [w814]
    tunnel: w233 -> [w813]
    shift-right: [w806] -> _
    shift-left: _ -> [w812]
    shift-right: [w811] -> _
    shift-left: u32 0 ("New Lost") -> [w805]
    shift-right: [w810] -> w45
    shift-left: u32[] [] ("NewBuffNum") -> [w801]
    shift-right: [w809] -> w48
    shift-left: u32[] [] ("NewNumLost") -> [w802]
    tunnel: w219 -> [w800]
    tunnel: w186 -> [w798]
    i -> [w793]
    stop <- w803 stop-if-true
    n203 = call <vilib>:"IMAQdx Get Image.vi"("Buffer Number Mode (Next)"=IMAQdx_Buffer_Number_Mode."Buffer Number", "error in"=w815, "Buffer Number In"=w793, "Image In"=w814, "Session In"=w816) -> ("error out"=w824:errorcluster, "Buffer Number Out"=w806:u32, "Image Out"=w795:T1, "Session Out"=w807:T4)  [unwired: 3 in]
    "Last Whisk\nBuffer 2" <- w806
    "?" <- w795
    n204 = Greater?(x=w793, y=w798) -> (0:→"Pupil Cam":bool)
    n205 = call "TrackPupilDroppedFrames_DALSA_IOS.vi"("NumLost"=w802, "BuffNum"=w801, "Curr Buffer"=w806, "Prev Lost"=w805, "Prev Buffer"=w812) -> ("New Lost"=w811:u32, "NewNumLost"=w809:u32[], "NewBuffNum"=w810:u32[])  [unwired: 4 in]
    "Dropped 2" <- w811
    n206 = call "IMAQ ImageToArray"("error in (no error)"=w824, "Image"=w795) -> ("error out"=w823:errorcluster, "Image Pixels (U8)"=w822:u8[][])  [unwired: 2 in, 3 out]
    n207 = Add(x=w806, y=w805) -> (x+y=w804:u32)
    n208 = Greater Or Equal?(x=w804, y=w800) -> ()  [unwired: 1 out]
    n209 = Write to Binary File(file (use dialog)=w813, data=w822, error in=w823, 5:FALSE ("prepend array or string size? (T)"), 9:T11."little-endian" ("byte order (0:big-endian, network order)")) -> (refnum out=w817:refnum<file>, error out=w808:errorcluster)  [unwired: 1 in, 1 out]
    n210 = local read "stop"() -> (w797:bool)
    n211 = local read "CBV Camera"() -> (w796:bool)
    n212 = call <vilib>:"Calculate Frames per Second.vi"("Update Interval (ms)"=u32 2000, "Buffer Number"=w806) -> ("Processed Frames/s"=→"Pupil Cam Fs":dbl)  [unwired: 7 in, 2 out]
    n213 = Unbundle By Name(w808) -> ("status"=w794:bool)
    n214 = Compound Arithmetic op=OR(w794, w797, w796) -> (w803:bool)
  }
  n215 = flat-sequence {
    tunnel: w103 -> [w869]
    tunnel: w102 -> [w868]
    tunnel: [w867] -> w101
    tunnel: [w866] -> w100
    tunnel: w99 -> [w865]
    tunnel: w98 -> [w864]
    tunnel: [w863] -> w97
    tunnel: [w862] -> w96
    tunnel: [w861] -> w94
    tunnel: w93 -> [w861]
    tunnel: w92 -> [w844]
    tunnel: [w844] -> w91
    tunnel: w87 -> [w860]
    tunnel: w86 -> [w843]
    tunnel: [w859] -> w85
    tunnel: [w858] -> w84
    tunnel: w83 -> [w857]
    tunnel: w82 -> [w856]
    tunnel: [w855] -> _
    tunnel: [w854] -> _
    tunnel: [w855] -> w81
    tunnel: [w854] -> w80
    tunnel: w79 -> [w852]
    tunnel: w78 -> [w853]
    tunnel: w77 -> [w851]
    tunnel: [w850] -> w76
    tunnel: w74 -> [w848]
    tunnel: w73 -> [w849]
    tunnel: [w848] -> w71
    tunnel: [w847] -> w70
    tunnel: w69 -> [w847]
    tunnel: w67 -> [w846]
    tunnel: [w846] -> w66
    tunnel: w64 -> [w845]
    tunnel: [w845] -> w63
    tunnel: [w844] -> w60
    tunnel: [w843] -> w59
    tunnel: w56 -> [w842]
    tunnel: [w842] -> w57
    tunnel: w54 -> [w841]
    tunnel: [w841] -> w53
    tunnel: w51 -> [w840]
    tunnel: [w840] -> w50
    tunnel: w48 -> [w839]
    tunnel: [w839] -> w47
    tunnel: w45 -> [w838]
    tunnel: [w838] -> w44
    tunnel: w42 -> [w837]
    tunnel: [w837] -> w41
    tunnel: w39 -> [w836]
    tunnel: [w836] -> w38
    tunnel: w35 -> [w835]
    tunnel: [w835] -> w34
    tunnel: w30 -> [w834]
    tunnel: [w834] -> w29
    tunnel: w25 -> [w833]
    tunnel: [w833] -> w24
    tunnel: [w829] -> w12
    tunnel: [w828] -> w11
    tunnel: w10 -> [w827]
    tunnel: w7 -> [w826]
    tunnel: w101 -> [w898]
    tunnel: w100 -> [w897]
    tunnel: w97 -> [w896]
    tunnel: w96 -> [w895]
    tunnel: w94 -> [w894]
    tunnel: w91 -> [w893]
    tunnel: w85 -> [w892]
    tunnel: w84 -> [w891]
    tunnel: w81 -> [w890]
    tunnel: w80 -> [w889]
    tunnel: w76 -> [w888]
    tunnel: [w888] -> w75
    tunnel: [w887] -> w72
    tunnel: w71 -> [w887]
    tunnel: w70 -> [w886]
    tunnel: [w886] -> w68
    tunnel: w66 -> [w885]
    tunnel: [w885] -> w65
    tunnel: w63 -> [w884]
    tunnel: [w884] -> w62
    tunnel: [w883] -> w61
    tunnel: w60 -> [w883]
    tunnel: w59 -> [w882]
    tunnel: [w882] -> w58
    tunnel: w57 -> [w881]
    tunnel: [w881] -> w55
    tunnel: w53 -> [w880]
    tunnel: [w880] -> w52
    tunnel: [w879] -> w49
    tunnel: w50 -> [w879]
    tunnel: w47 -> [w878]
    tunnel: [w878] -> w46
    tunnel: w44 -> [w877]
    tunnel: [w877] -> w43
    tunnel: w41 -> [w876]
    tunnel: [w876] -> w40
    tunnel: w38 -> [w875]
    tunnel: [w875] -> w37
    tunnel: w34 -> [w874]
    tunnel: [w874] -> w32
    tunnel: w29 -> [w873]
    tunnel: [w873] -> w27
    tunnel: [w872] -> w26
    tunnel: w24 -> [w872]
    tunnel: w12 -> [w871]
    tunnel: w11 -> [w870]
    frame #0 {
      n216 = call-poly <vilib>:"DAQmx Write.vi"("task/channels in"=w827, "data"=FALSE, "error in"=w826) -> ("task out"=w831:refnum<k21>, "error out"=w832:errorcluster)  [unwired: 10 in, 1 out]
      n217 = call <vilib>:"DAQmx Stop Task.vi"("task/channels in"=w869, "error in"=w868) -> ("task out"=w867:refnum<k21>, "error out"=w866:errorcluster)  [unwired: 12 in]
      n218 = call <vilib>:"DAQmx Stop Task.vi"("task/channels in"=w865, "error in"=w864) -> ("task out"=w863:refnum<k21>, "error out"=w862:errorcluster)  [unwired: 12 in]
      n219 = call <vilib>:"DAQmx Stop Task.vi"("task/channels in"=w857, "error in"=w856) -> ("task out"=w855:refnum<k21>, "error out"=w854:errorcluster)  [unwired: 12 in]
      n220 = call <vilib>:"IMAQdx Close Camera.vi"("error in"=w848, "Session In"=w849) -> ()  [unwired: 9 in, 1 out]
      n221 = call "IMAQ AVI2 Close"("error in (no error)"=w852, "AVI Refnum"=w851) -> ("error out"=w850:errorcluster)  [unwired: 9 in]
      n222 = call <vilib>:"IMAQdx Close Camera.vi"("error in"=w852, "Session In"=w853) -> ()  [unwired: 9 in, 1 out]
      n223 = call <vilib>:"DAQmx Stop Task.vi"("task/channels in"=w860, "error in"=w843) -> ("task out"=w859:refnum<k21>, "error out"=w858:errorcluster)  [unwired: 12 in]
      n224 = call <vilib>:"DAQmx Stop Task.vi"("task/channels in"=w831, "error in"=w832) -> ("task out"=w829:refnum<k21>, "error out"=w828:errorcluster)  [unwired: 12 in]
    }
    frame #1 {
      n225 = call <vilib>:"DAQmx Clear Task.vi"("task in"=w871, "error in"=w870) -> ()  [unwired: 13 in, 1 out]
      n226 = call <vilib>:"DAQmx Clear Task.vi"("task in"=w898, "error in"=w897) -> ()  [unwired: 13 in, 1 out]
      n227 = call <vilib>:"DAQmx Clear Task.vi"("task in"=w896, "error in"=w895) -> ()  [unwired: 13 in, 1 out]
      n228 = call <vilib>:"IMAQdx Close Camera.vi"("error in"=w893, "Session In"=w894) -> ()  [unwired: 9 in, 1 out]
      n229 = call <vilib>:"DAQmx Clear Task.vi"("task in"=w890, "error in"=w889) -> ()  [unwired: 13 in, 1 out]
      n230 = call <vilib>:"DAQmx Clear Task.vi"("task in"=w892, "error in"=w891) -> ()  [unwired: 13 in, 1 out]
    }
  }
  n231 = call <vilib>:"IMAQ Extract Buffer.vi"("error in (no error)"=w37, "Buffer to extract"=-1, "IMAQ Session In"=w40) -> ("error out"=w476:errorcluster, "IMAQ Session Out"=w475:refnum<k11>)  [unwired: 7 out]
  n232 = Close File(refnum=w65, error in=w58) -> (path=w375:path)  [unwired: 1 out]
  n233 = Delete From Array(array=w49, length=1, index=0) -> (array with subset deleted=w280:u32[])  [unwired: 1 out]
  n234 = Delete From Array(array=w52, length=1, index=0) -> (array with subset deleted=w281:u32[])  [unwired: 1 out]
  n235 = Delete From Array(array=w46, length=1, index=0) -> (array with subset deleted=w206:u32[])  [unwired: 1 out]
  n236 = Delete From Array(array=w43, length=1, index=0) -> (array with subset deleted=w205:u32[])  [unwired: 1 out]
  n237 = Close File(refnum=w68, error in=w72) -> (path=w374:path, error out=w373:errorcluster)
  n238 = Close File(refnum=w62, error in=w61) -> (path=w202:path, error out=w201:errorcluster)
  n239 = Build Array(w280, w281) -> (w283:u32[][])
  n240 = call <vilib>:"IMAQ Close.vi"("error in (no error)"=w476, "IMAQ Session In"=w475) -> ("error out"=w477:errorcluster)  [unwired: 9 out]
  n241 = Build Array(w205, w206) -> (w208:u32[][])
  n242 = Array To Spreadsheet String(delimiter (Tab)=",", array=w281, 3:"%d" ("format string")) -> (spreadsheet string=w298:string)
  n243 = Transpose 2D Array(2D array=w283) -> (transposed array=w282:u32[][])
  n244 = Array To Spreadsheet String(delimiter (Tab)=",", array=w280, 3:"%d" ("format string")) -> (spreadsheet string=w299:string)
  n245 = Move(source path=w202, error in=w201, 10:"Target Path") -> (error out=w203:errorcluster)  [unwired: 2 in, 2 out]
  n246 = Move(source path=w374, error in=w373, 10:"Target Path") -> (error out=w371:errorcluster)  [unwired: 2 in, 2 out]
  n247 = Array To Spreadsheet String(delimiter (Tab)=",", array=w206, 3:"%d" ("format string")) -> (spreadsheet string=w209:string)
  n248 = Transpose 2D Array(2D array=w208) -> (transposed array=w207:u32[][])
  n249 = Move(source path=w26, error in=w75, 10:"Target Path") -> (error out=w370:errorcluster)  [unwired: 2 in, 2 out]
  n250 = Array To Spreadsheet String(delimiter (Tab)=",", array=w205, 3:"%d" ("format string")) -> (spreadsheet string=w210:string)
  n251 = for {
    N: w27 -> [_]
    tunnel: w32 -> [w902] mode=indexing
    shift-right: [w900] -> w377
    shift-left: w477 -> [w901]
    n252 = call "IMAQ Dispose"("All Images? (No)"=FALSE, "Image"=w902, "error in (no error)"=w901) -> ("error out"=w900:errorcluster)  [unwired: 3 out]
  }
  n253 = call <vilib>:"Trim Whitespace.vi"("string"=w299) -> ("trimmed string"=w195:string)  [unwired: 1 in]
  n254 = call <vilib>:"Trim Whitespace.vi"("string"=w298) -> ("trimmed string"=w194:string)  [unwired: 1 in]
  n255 = Number To Decimal String(number=w282) -> ()  [unwired: 1 in, 1 out]
  n256 = call <vilib>:"Trim Whitespace.vi"("string"=w210) -> ("trimmed string"=w196:string)  [unwired: 1 in]
  n257 = call <vilib>:"Trim Whitespace.vi"("string"=w209) -> ("trimmed string"=w197:string)  [unwired: 1 in]
  n258 = Number To Decimal String(number=w207) -> ()  [unwired: 1 in, 1 out]
  n259 = call <vilib>:"Simple Error Handler.vi"("error in (no error)"=w203) -> ()  [unwired: 1 in, 8 out]
  n260 = call <vilib>:"Simple Error Handler.vi"("error in (no error)"=w371) -> ()  [unwired: 1 in, 8 out]
  n261 = call <vilib>:"Simple Error Handler.vi"("error in (no error)"=w370) -> ()  [unwired: 1 in, 8 out]
  n262 = Build Array(w196, w197, w195, w194) -> (w193:string[])
  n263 = Move(source path=w375, error in=w377, 10:"Target Path") -> (error out=w376:errorcluster)  [unwired: 2 in, 2 out]
  n264 = TDMS Set Properties(5:w193, 7:string[] ["PupilCam_DroppedFrameIndex", "PupilCam_NumberDropped", "WhiskCam_DroppedFrameIndex", "WhiskCam_NumberDropped"] ("channel name(s) in (Untitled)"), 8:w58, 11:w55) -> (0:w305:errorcluster, 3:w304:refnum<k34>)  [unwired: 2 in, 2 out]
  n265 = TDMS Close(8:w305, 11:w304) -> (0:w378:errorcluster, 3:w367:path)
  n266 = Path To String(path=w367) -> (string=w369:string)
  n267 = call <vilib>:"Simple Error Handler.vi"("error in (no error)"=w376) -> ()  [unwired: 1 in, 8 out]
  n268 = TDMS Defragment(4:w378, 7:w367) -> (0:w364:errorcluster)
  n269 = Concatenate Strings(w369, "_index" ("string")) -> (w366:string)
  n270 = String To Path(string=w366) -> (path=w365:path)
  n271 = Move(source path=w367, error in=w364, 10:"Target Path") -> (error out=w372:errorcluster)  [unwired: 2 in, 2 out]
  n272 = Move(source path=w365, error in=w364, 10:"Target Path") -> (error out=w204:errorcluster)  [unwired: 2 in, 2 out]
  n273 = call <vilib>:"Simple Error Handler.vi"("error in (no error)"=w372) -> ()  [unwired: 1 in, 8 out]
  n274 = call <vilib>:"Simple Error Handler.vi"("error in (no error)"=w204) -> ()  [unwired: 1 in, 8 out]
